vi "RP Transceiver Test.vi"() -> ()   [LabVIEW 2016]
uses:
  RP Transceiver.lvclass
  Receiver format.ctl
panel:
  in  "Step":dbl
  in  "End":dbl
  in  "Start":dbl
  in  "Server address":string="192.168.1.100"
  in  "Averaging time":dbl format="%#_6p"
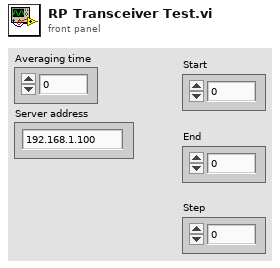
[diagram p1: front panel]
types:
  T1 = typedef "Receiver format.ctl" = enum16{"X-Y-F", "F-X-Y", "X-Y", "X"}
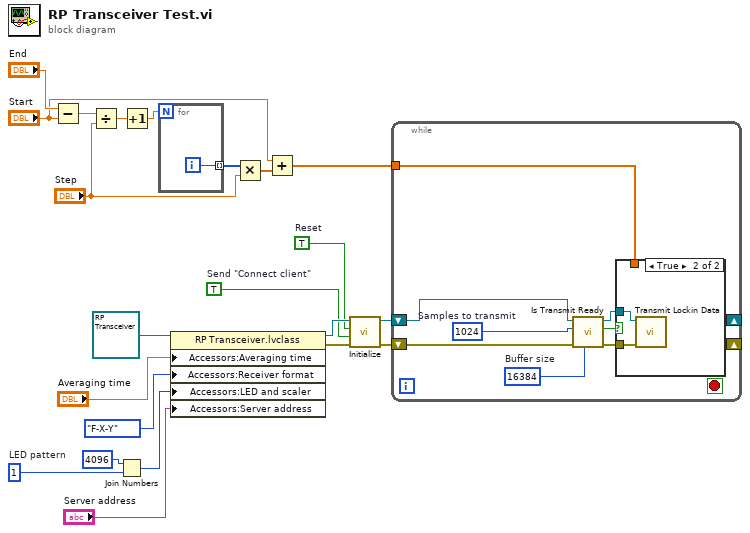
[diagram p0: block diagram]
diagram:
  w12 = TRUE  # Send "Connect client"
  w13 = TRUE  # Reset
  w17 = i16 1  # LED pattern
  n1 = Subtract(x="End", y="Start") -> (x-y=w8:dbl)
  n2 = Divide(x=w8, y="Step") -> (x/y=w7:dbl)
  n3 = Join Numbers(hi=i16 4096, lo=w17) -> ((hi.lo)=w19:u32)
  n4 = Increment(x=w7) -> (x+1=w6:dbl)
  n5 = for {
    N: w6 -> [_]
    tunnel: [w23] -> w5 mode=indexing
    i -> [w23]
  }
  n6 = property class="RP Transceiver.lvclass"(reference=refnum<class "RP Transceiver.lvclass"> refnum ("RP Transceiver.lvclass"), "Accessors:Averaging time"="Averaging time", "Accessors:Receiver format"=Receiver_format."F-X-Y" ("Receiver format"), "Accessors:LED and scaler"=w19, "Accessors:Server address"="Server address") -> (reference out=w15:refnum<class "RP Transceiver.lvclass">, error out=w14:errorcluster)  [unwired: 1 in]
  n7 = Multiply(x=w5, y="Step") -> (x*y=w3:dbl[])
  n8 = Add(x="Start", y=w3) -> (x+y=w1:dbl[])
  n9 = call-dynamic "Initialize.vi"("error in (no error)"=w14, "Send \"Connect client\""=w12, "Reset"=w13, "RP Transceiver in"=w15) -> ("error out"=w10:errorcluster, "RP Transceiver out"=w11:refnum<class "RP Transceiver.lvclass">)  [unwired: 6 in]
  n10 = while {
    shift-right: _ -> [_]
    shift-left: w11 -> [w28]
    shift-right: _ -> [_]
    shift-left: w10 -> [w31]
    tunnel: w1 -> [w24]
    stop <- _ stop-if-true
    w29 = 1024  # Samples to transmit
    w30 = 16384  # Buffer size
    n11 = call-dynamic "Is Transmit Ready.vi"("Buffer size"=w30, "error in (no error)"=w31, "Samples to transmit"=w29, "RP Instrument in"=w28) -> ("error out"=w26:errorcluster, "Transmit Ready"=w27:bool, "RP Instrument out"=w25:refnum<class "RP Transceiver.lvclass">)  [unwired: 4 in, 1 out]
    n12 = case shown="True" w27 {
      tunnel: w26 -> [_ w33]
      tunnel: w25 -> [_ w32]
      tunnel: w24 -> [_ _]
      frame False {
      }
      frame True {
        n13 = call-dynamic "Transmit Lockin Data.vi"("error in (no error)"=w33, "RP Transceiver in"=w32) -> ()  [unwired: 7 in, 3 out]
      }
    }
  }
